vi "Insert Test Step.vi"(8 "error in (no error)":errorcluster, 10 "Insert Test Step":T1, 11 "Process Builder Model in":refnum<class "Process Builder Model.lvclass">) -> (0 "error out":errorcluster, 3 "Process Builder Model out":refnum<class "Process Builder Model.lvclass">, 5 "Unique ID out":string)   [LabVIEW 2019, in "Process Builder Model.lvclass"]
uses:
  <vilib>/gpm_packages/@cs/Car-wash/Source/Process Builder Model/Process Builder Model.lvclass
  C:/Program Files/National Instruments/LabVIEW 2019/vi.lib/gpm_packages/@cs/Test-executive-builder/Source/Test Executive Builder Model/Test Executive Builder Model/Test Executive Builder Model.lvclass
  C:/Program Files/National Instruments/LabVIEW 2019/vi.lib/ActorFramework/Actor/Actor.lvclass
  <vilib>/gpm_packages/@cs/Test-executive-builder/Source/Application Dependencies/Insert Test Step.ctl
  <vilib>/gpm_packages/@cs/Car-wash/Source/iProcess Step Model/iProcess Step Model/iProcess Step Model.lvclass
  <vilib>/gpm_packages/@cs/Test-executive-builder/Source/Test Executive Builder Model/Test Executive Builder Model/Test Executive Builder Model.lvclass/Test Executive Builder Model.ctl
  <vilib>/ActorFramework/Actor/Actor.lvclass/Actor.ctl
  <vilib>/ActorFramework/Message Enqueuer/Message Enqueuer.lvclass/Message Enqueuer.ctl
  <vilib>/ActorFramework/Message Enqueuer/Init from Existing Queue.vi
  <vilib>/ActorFramework/Message Enqueuer/Enqueue.vi
  <vilib>/gpm_packages/@cs/Test-executive-builder/Source/Test Executive Builder Model/Test Executive Builder Model Messages/Redraw Tree Msg/Redraw Tree Msg.lvclass
  C:/Program Files/National Instruments/LabVIEW 2019/vi.lib/ActorFramework/Message/Message.lvclass
  <vilib>/ActorFramework/Message Priority Queue/Priority Enqueue.vi
  <vilib>/ActorFramework/Message Enqueuer/Message Enqueuer.lvclass
  <vilib>/gpm_packages/@cs/Test-executive-builder/Source/Test Executive Builder Model/Test Executive Builder Model/Test Executive Builder Model.lvclass
  <vilib>/gpm_packages/@cs/test-executive/Source/Test Executive/Executioner/Executioner.lvclass
  <vilib>/gpm_packages/@cs/test-executive/Source/Test Executive/TestExecutive Ref/TestExecutive Ref.lvclass
  <vilib>/ActorFramework/Actor/Actor.lvclass
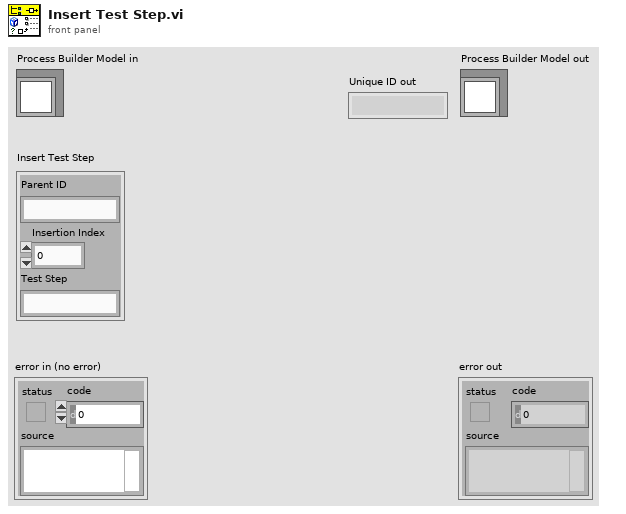
[diagram p1: front panel]
types:
  T1 = typedef "Insert Test Step.ctl" = cluster{"Parent ID":string, "Insertion Index":i32, "Test Step":string}
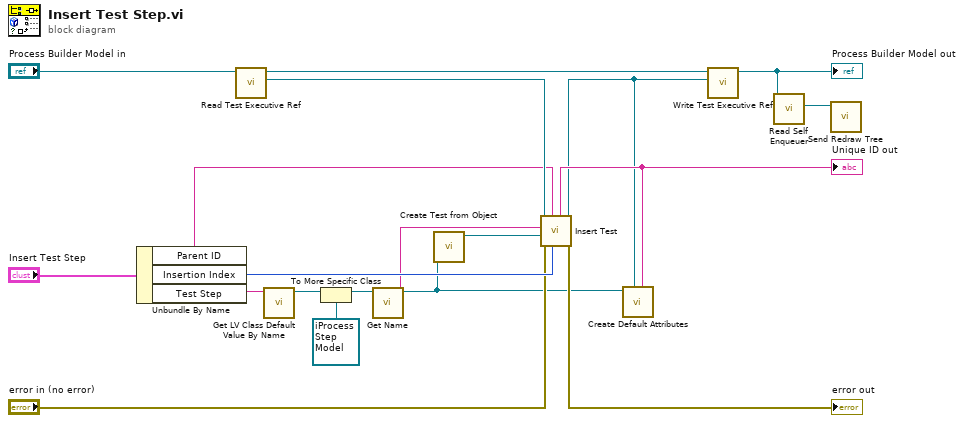
[diagram p0: block diagram]
diagram:
  n1 = Unbundle By Name("Insert Test Step") -> ("Parent ID"=w11:string, "Insertion Index"=w9:i32, "Test Step"=w16:string)
  n2 = call <vilib>:"Read Test Executive Ref.vi"("Test Executive Builder Model in"="Process Builder Model in") -> ("Test Executive Ref"=w12:refnum<data-value>, "Test Executive Builder Model out"=w18:refnum<class "Process Builder Model.lvclass">)  [unwired: 9 in]
  n3 = call <vilib>:"Get LV Class Default Value By Name.vi"("class name"=w16) -> ("object"=w15:refnum<class>)  [unwired: 9 in, 1 out]
  n4 = To More Specific Class(target class=refnum<class "iProcess Step Model.lvclass"> refnum ("iProcess Step Model.lvclass"), reference=w15) -> (specific class reference=w13:refnum<class "iProcess Step Model.lvclass">)  [unwired: 1 in, 1 out]
  n5 = call <vilib>:"Get Name.vi"("iProcess Step Model in"=w13) -> ("Name"=w8:string, "iProcess Step Model out"=w3:refnum<class "iProcess Step Model.lvclass">)  [unwired: 9 in]
  n6 = call <vilib>:"Create Test from Object.vi"("Test"=w3) -> ("Test"=w10:refnum<class "Executioner.lvclass">)  [unwired: 10 in]
  n7 = call <vilib>:"Insert Test.vi"("Insertion Index"=w9, "Parent ID"=w11, "error in (no error)"="error in (no error)", "Test"=w10, "Name"=w8, "Test Executive Ref"=w12) -> ("error out"=→"error out":errorcluster, "Test Executive Ref out"=w1:refnum<data-value>, "Unique ID out"=w2:string)  [unwired: 2 in, 1 out]
  "Unique ID out" <- w2
  n8 = call-dynamic "Create Default Attributes.vi"("Unique ID"=w2, "Process Executive Ref"=w1, "iProcess Step Model in"=w3) -> ()  [unwired: 8 in, 1 out]
  n9 = call <vilib>:"Write Test Executive Ref.vi"("Test Executive Ref"=w1, "Test Executive Builder Model in"=w18) -> ("Test Executive Builder Model out"=w5:refnum<class "Process Builder Model.lvclass">)  [unwired: 9 in]
  "Process Builder Model out" <- w5
  n10 = call <vilib>:"Read Self Enqueuer.vi"("Actor"=w5) -> ("Self Enqueuer"=w4:refnum<class "Message Enqueuer.lvclass">)  [unwired: 10 in]
  n11 = call <vilib>:"Send Redraw Tree.vi"("Message Enqueuer"=w4) -> ()  [unwired: 9 in, 2 out]
